vi "ECU.vi"() -> ()   [LabVIEW 2017]
panel:
  out "?":ext
  out "?":ext
  out "?":ext
  out "?":ext
  out "?":ext
  out "?":ext
  out "Check Engine":bool
  in  "Failure throttle \nPosition Sensor":bool
  in  "Lack of signal rotational\n speed":bool
  out "Injection time(ms)":dbl
  in  "Throttle Position(deg )":dbl(knob) scale=0.0..10.0
  out "Injection time after correction (us)":dbl
  in  "Lack of signal oxygen \nSensor":bool
  in  "Oxygen Sensor [V]":dbl(knob) scale=0.2..1.2
  out "Injection time after voltage and temperature correction(us)":dbl
  in  "Voltage Supply[V]":dbl(knob) scale=0.0..15.0
  in  "Temparature Cooling Liquid\nTemparature Sensor":bool
  in  "Temparature Correction":dbl[](array[numeric])
  out "Injection time after temparature correction(ms)":dbl
  in  "Cooling Liquid Temparature(degree)":dbl(slide) scale=-20.0..120.0
  in  "?":dbl[][](array[numeric])
  out "Basic Injection time(ms)":dbl format="%.0g"
  in  "Pressure in the suction manifold":dbl(slide) scale=0.0..90.0
  in  "Engine Rotational Speed(rpm)":dbl(knob) scale=800.0..2600.0
  in  "?":bool
  # "ECU MEMORY"
  # "-20"
  # "0"
  # "20"
  # "40"
  # "60"
  # "80"
  # "100"
  # "120"
  # "Cooling Liquid Temperature"
  # "Basic Engine Map"
  # "0"
  # "10"
  # "20"
  # "30"
  # "40"
  # "50"
  # "60"
  # "70"
  # "80"
  # "90"
  # "Engine Rotational Speed"
  # "800"
  # "Absolute pressure in \nthe sunction manifold"
  # "1000"
  # "1200"
  # "1400"
  # "1600"
  # "1800"
  # "2000"
  # "2200"
  # "2400"
  # "2600"
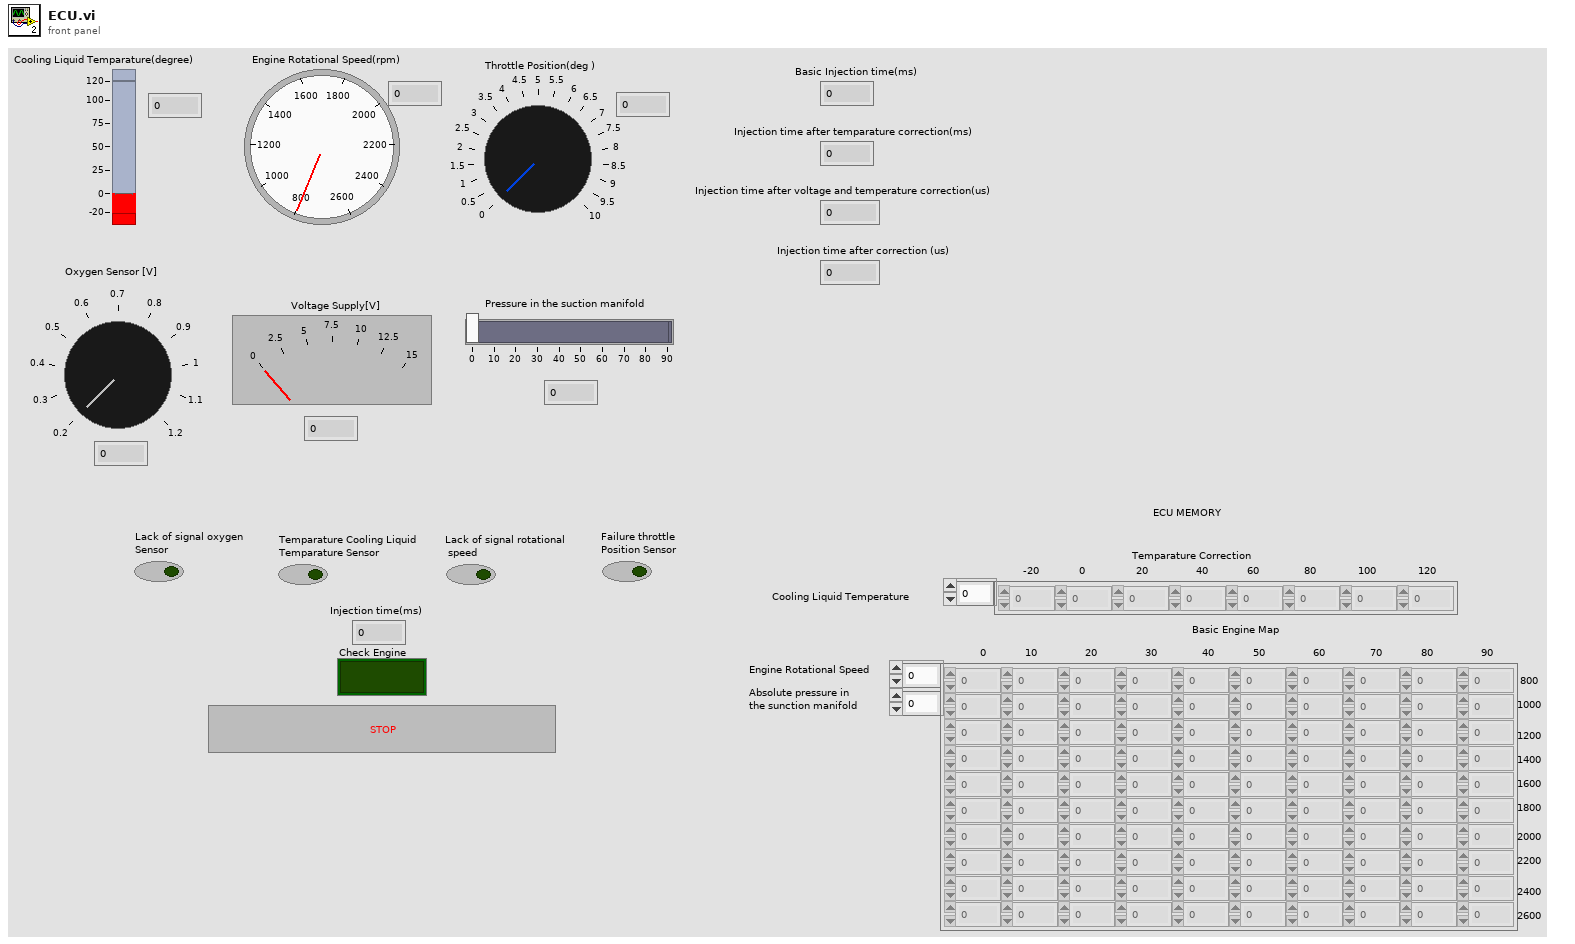
[diagram p1: front panel]
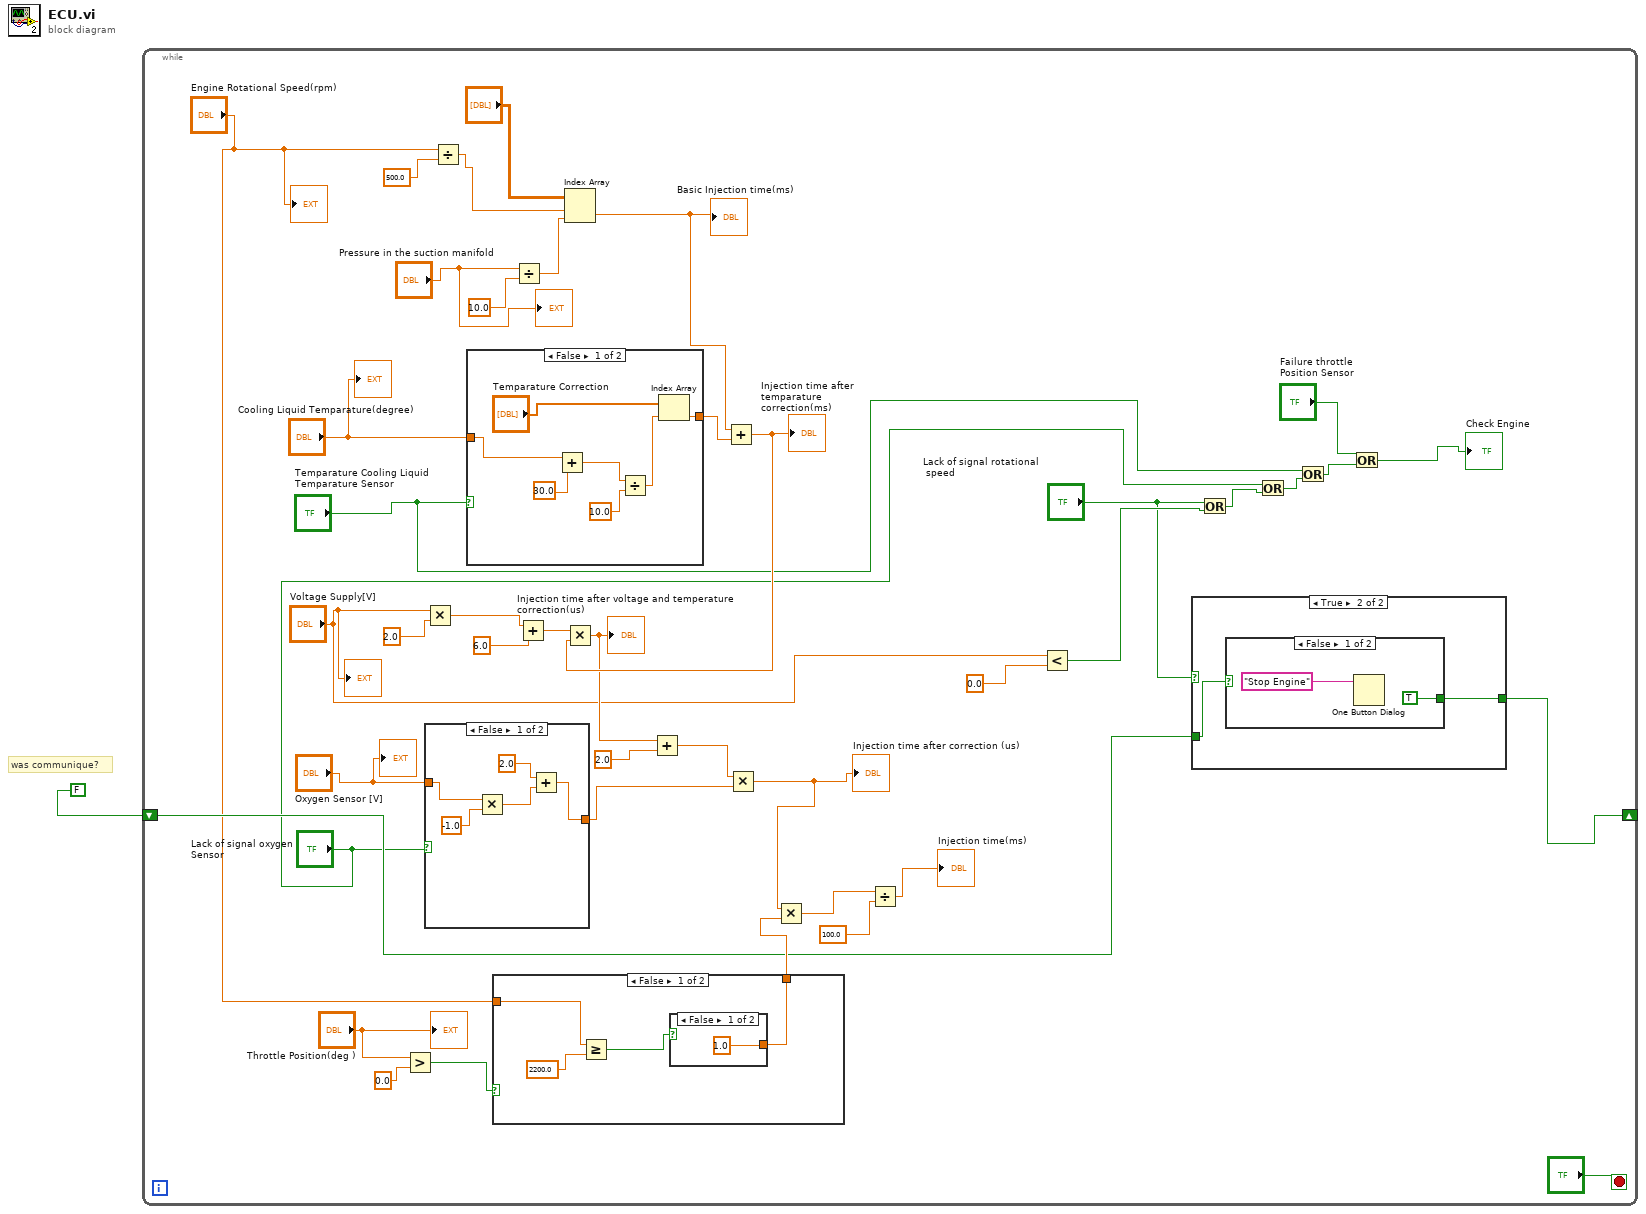
[diagram p0: block diagram]
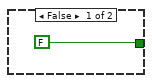
[diagram p2: hidden frame]
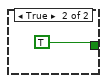
[diagram p3: hidden frame]
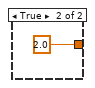
[diagram p6: hidden frame]
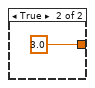
[diagram p7: hidden frame]
diagram:
  # "was communique?"
  n1 = while {
    shift-right: [w25] -> _
    shift-left: FALSE -> [w26]
    stop <- "?" stop-if-true
    n2 = Greater?(x="Throttle Position(deg )", y=0.0) -> (0:w31:bool)
    n3 = Multiply(x="Voltage Supply[V]", y=2.0 ("Numeric")) -> (x*y=w39:dbl)
    n4 = case shown="False" "Lack of signal oxygen \nSensor" {
      tunnel: "Oxygen Sensor [V]" -> [w59 _]
      tunnel: [w57 2.0] -> w35
      frame False {
        n5 = Multiply(x=w59, y=-1.0) -> (x*y=w58:dbl)
        n6 = Add(x=2.0, y=w58) -> (x+y=w57:dbl)
      }
      frame True {
      }
    }
    n7 = Divide(x="Engine Rotational Speed(rpm)", y=500.0) -> (x/y=w15:dbl)
    n8 = case shown="False" "Temparature Cooling Liquid\nTemparature Sensor" {
      tunnel: "Cooling Liquid Temparature(degree)" -> [w64 _]
      tunnel: [w61 3.0] -> w40
      frame False {
        n9 = Add(x=w64, y=30.0) -> (x+y=w65:dbl)
        n10 = Divide(x=w65, y=10.0) -> (x/y=w66:dbl)
        n11 = Index Array(array="Temparature Correction", index=w66) -> (element=w61:dbl)
      }
      frame True {
      }
    }
    n12 = case shown="False" w31 {
      tunnel: "Engine Rotational Speed(rpm)" -> [w53 _]
      tunnel: [w50 _] -> w28
      frame False {
        n13 = Greater Or Equal?(x=w53, y=2200.0) -> (x >= y?=w51:bool)
        n14 = case shown="False" w51 {
          tunnel: [1.0 _] -> w50
          frame False {
          }
          frame True {
          }
        }
      }
      frame True {
      }
    }
    n15 = Divide(x="Pressure in the suction manifold", y=10.0) -> (x/y=w13:dbl)
    n16 = Add(x=w39, y=6.0) -> (x+y=w38:dbl)
    n17 = Index Array(array="?", index (row)=w15, index (col)=w13) -> (element=w12:dbl)
    "Basic Injection time(ms)" <- w12
    n18 = Add(x=w12, y=w40) -> (x+y=w36:dbl)
    "Injection time after temparature correction(ms)" <- w36
    n19 = Multiply(x=w38, y=w36) -> (x*y=w33:dbl)
    "Injection time after voltage and temperature correction(us)" <- w33
    n20 = Add(x=w33, y=2.0) -> (x+y=w34:dbl)
    n21 = Multiply(x=w34, y=w35) -> (x*y=w29:dbl)
    "Injection time after correction (us)" <- w29
    n22 = Multiply(x=w29, y=w28) -> (x*y=w3:dbl)
    n23 = Divide(x=w3, y=100.0) -> (x/y=→"Injection time(ms)":dbl)
    n24 = Less?(x="Voltage Supply[V]", y=0.0) -> (x < y?=w24:bool)
    n25 = case shown="True" "Lack of signal rotational\n speed" {
      tunnel: w26 -> [_ w45]
      tunnel: [FALSE w46] -> w25
      frame False {
      }
      frame True {
        n26 = case shown="False" w45 {
          tunnel: [TRUE TRUE] -> w46
          frame False {
            n27 = One Button Dialog(message="Stop Engine") -> ()  [unwired: 1 in, 1 out]
          }
          frame True {
          }
        }
      }
    }
    n28 = Or(x="Lack of signal rotational\n speed", y=w24) -> (x .or. y?=w19:bool)
    n29 = Or(x="Lack of signal oxygen \nSensor", y=w19) -> (x .or. y?=w20:bool)
    n30 = Or(x="Temparature Cooling Liquid\nTemparature Sensor", y=w20) -> (x .or. y?=w21:bool)
    n31 = Or(x="Failure throttle \nPosition Sensor", y=w21) -> (x .or. y?=→"Check Engine":bool)
    "?" <- "Cooling Liquid Temparature(degree)"
    "?" <- "Engine Rotational Speed(rpm)"
    "?" <- "Voltage Supply[V]"
    "?" <- "Oxygen Sensor [V]"
    "?" <- "Pressure in the suction manifold"
    "?" <- "Throttle Position(deg )"
  }
